vi "mainSynchro_PIV_LAT_translation.vi"() -> ()   [LabVIEW 2023]
uses:
  sousVis/configUtilisateur.ctl
  sousVis/customParam.ctl
  sousVis/configFPGA.ctl
  sousVis/defaultParam.ctl
  <vilib>/Instr/_visa.llb/VISA Configure Serial Port (Instr).vi
panel:
  in  "Home":bool
  in  "Tab Control":T1(tab)
  in  "TestComMoteur":bool
  in  "ComControler":refnum<visa-resource-name> caption="Port Com contrôleur"
  in  "ComMoteur":refnum<visa-resource-name> caption="Port Com moteur translation"
  in  "WriteConf":bool
  in  "readConf":bool
  in  "Configuration Moteurs":T2
  in  "Configuration contrôleur":T3={"Nombre de période"=0, "Fréquence "=10, "Nb pulse préchauffe laser"=0, "skip_frame_PIV"=0, "skip_frame_LAT"=0, "Time beetwen pulses (µs)"=10000, "Temps LAT (µs)"=20000, "Temps expo LAT (µs)"=10000, "action"=enum."PIV"}
  in  "customParam":T4={"CamDelayToOpen(µs)"=10, "FLWidth(µs)"=10, "QSWidth(µs)"=10, "DelayFL_QS (µs)"=180, "CamDelayToClose(µs)"=100, "CamPivExposure(µs)"=100}
  in  "StopPIV":bool
  in  "Play Button":bool
  out "XY Graph":cluster{cluster{"t_periode":i32, dbl}[]}[](graph)
  out "error out":errorcluster
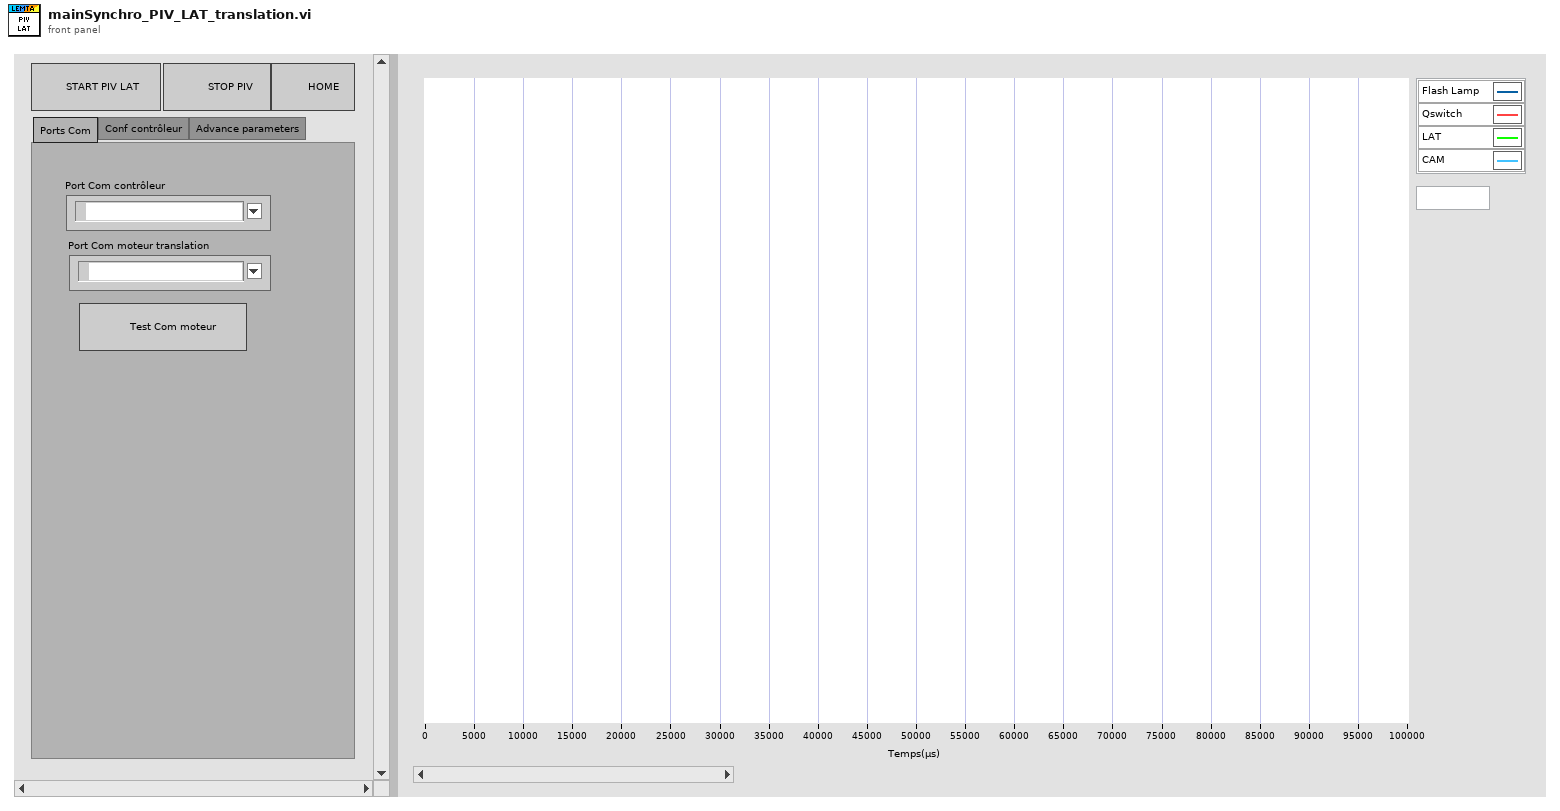
[diagram p1: front panel]
types:
  T1 = enum32{"Ports Com", "Conf contrôleur", "Advance parameters"}
  T2 = cluster{"Délais démarrage (ms)":dbl, "Vitesse (mm/s)":dbl, "Déplacement (mm)":dbl}
  T3 = typedef "configUtilisateur.ctl" = cluster{"Nombre de période":u16, "Fréquence ":u16, "Nb pulse préchauffe laser":u16, "skip_frame_PIV":u8, "skip_frame_LAT":u8, "Time beetwen pulses (µs)":u32, "Temps LAT (µs)":u32, "Temps expo LAT (µs)":u32, "action":enum8{"PIV", "PIV + LAT", "LAT"}}
  T4 = typedef "customParam.ctl" = cluster{"CamDelayToOpen(µs)":u32, "FLWidth(µs)":u32, "QSWidth(µs)":u32, "DelayFL_QS (µs)":u32, "CamDelayToClose(µs)":u32, "CamPivExposure(µs)":u32}
  T5 = typedef "configFPGA.ctl" = cluster{"action":enum8{"PIV", "PIV + LAT", "LAT", "STOP"}, "nb_periodes":u16, "t_periode":u32, "nb_pulse_prechauffe":u8, "nb_skip_frame_PIV":u8, "nb_skip_frame_LAT":u8, "t_FL1_start":u32, "t_FL1_stop":u32, "t_QS1_start":u32, "t_QS1_stop":u32, "t_FL2_start":u32, "t_FL2_stop":u32, "t_QS2_start":u32, "t_QS2_stop":u32, "t_LAT_start":u32, "t_LAT_stop":u32, "t_FRAME1_start":u32, "t_FRAME1_stop":u32, "t_FRAME2_start":u32, "t_FRAME2_stop":u32}
  T6 = typedef "defaultParam.ctl" = cluster{"customParam":T4, "Configuration":T3}
  T7 = cluster{"temps attente (ms)":i32, "vitesse (mm/s)":dbl, "Distance (mm)":dbl}
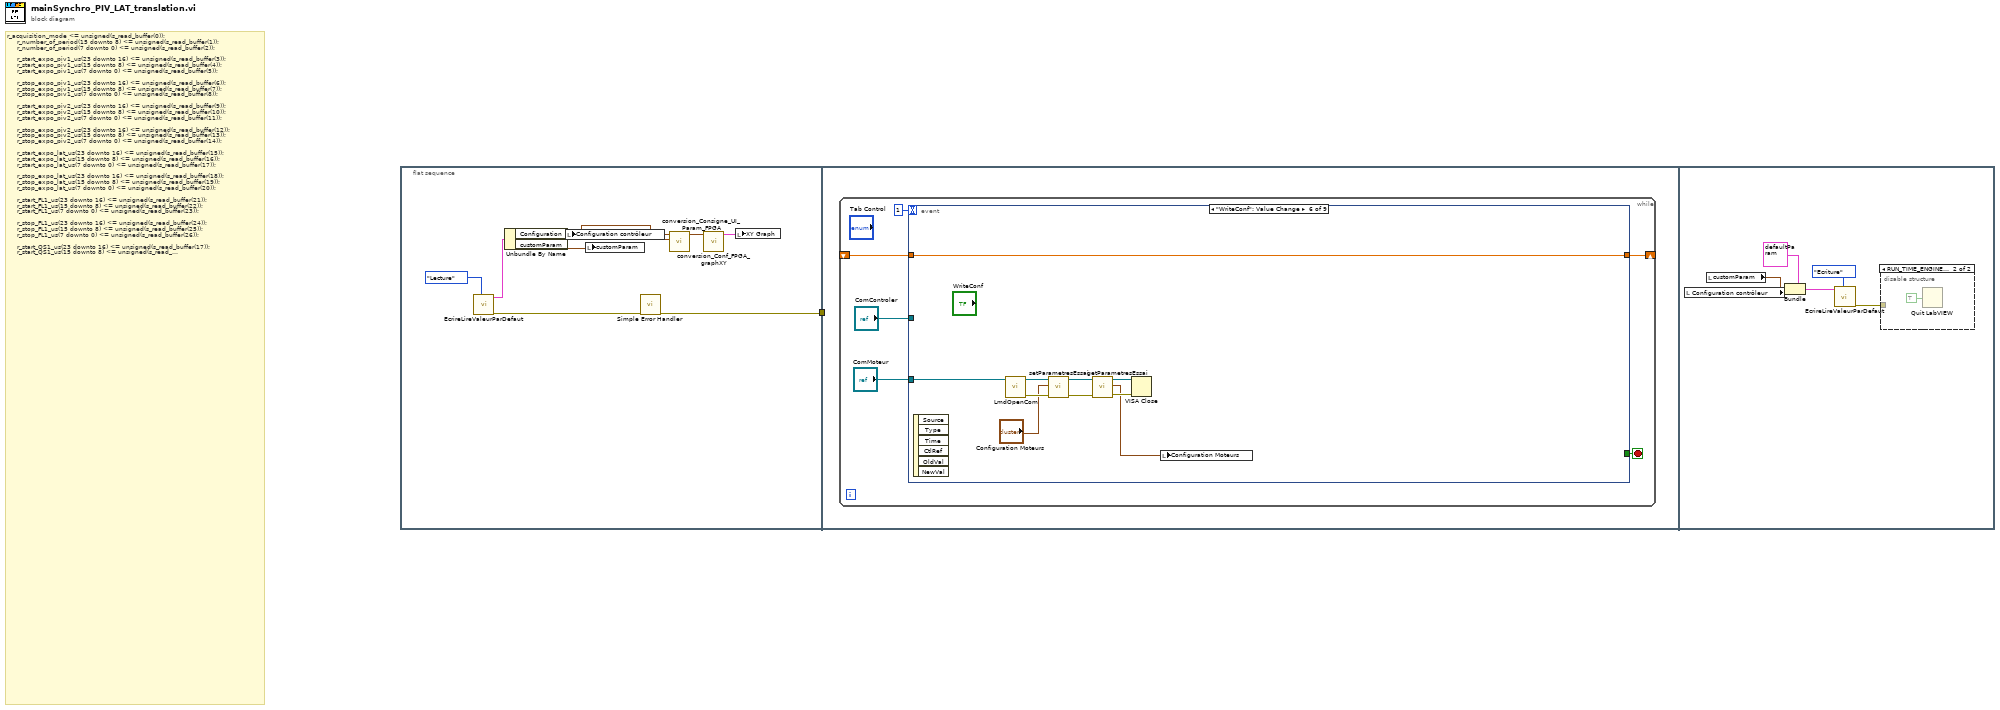
[diagram p0: block diagram]
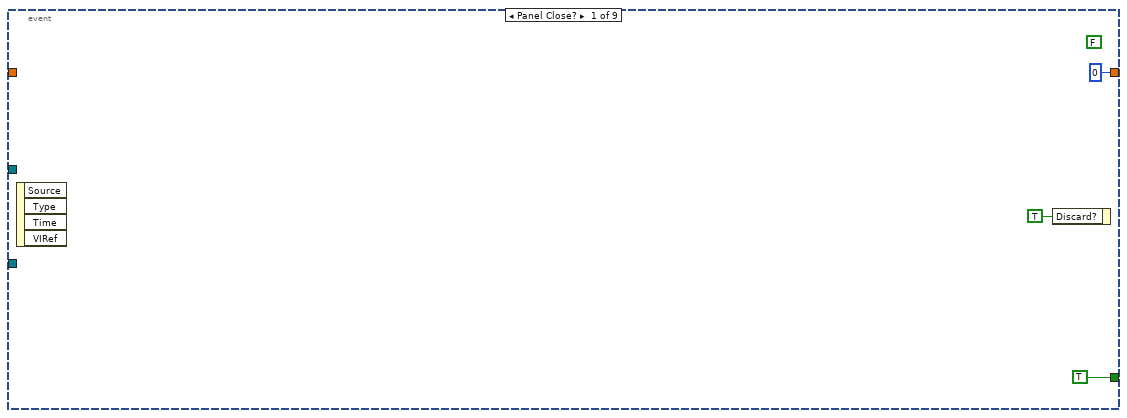
[diagram p2: hidden frame]
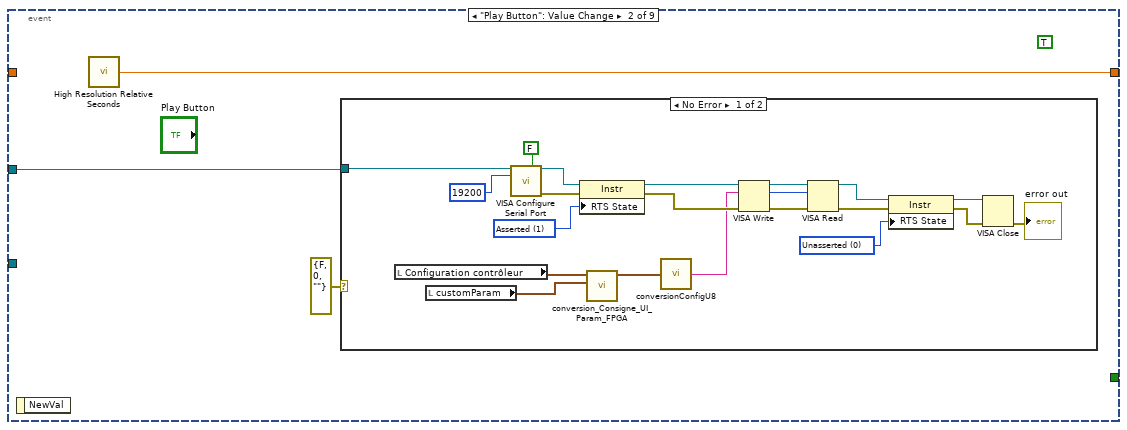
[diagram p3: hidden frame]
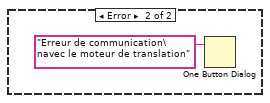
[diagram p4: hidden frame]
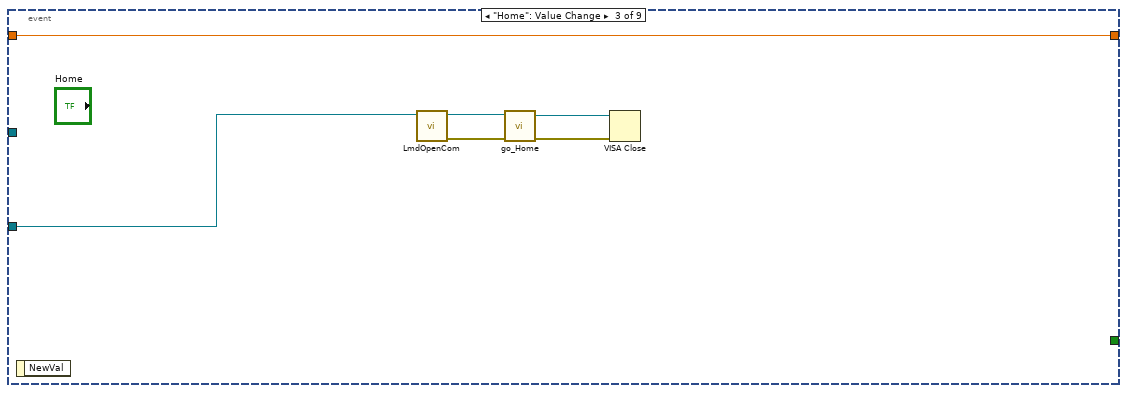
[diagram p5: hidden frame]
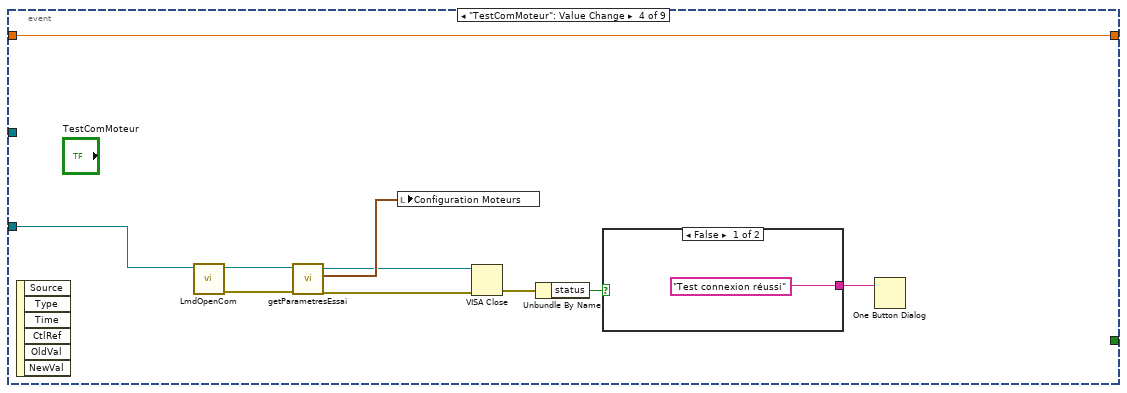
[diagram p6: hidden frame]
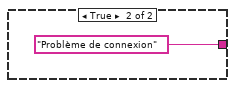
[diagram p7: hidden frame]
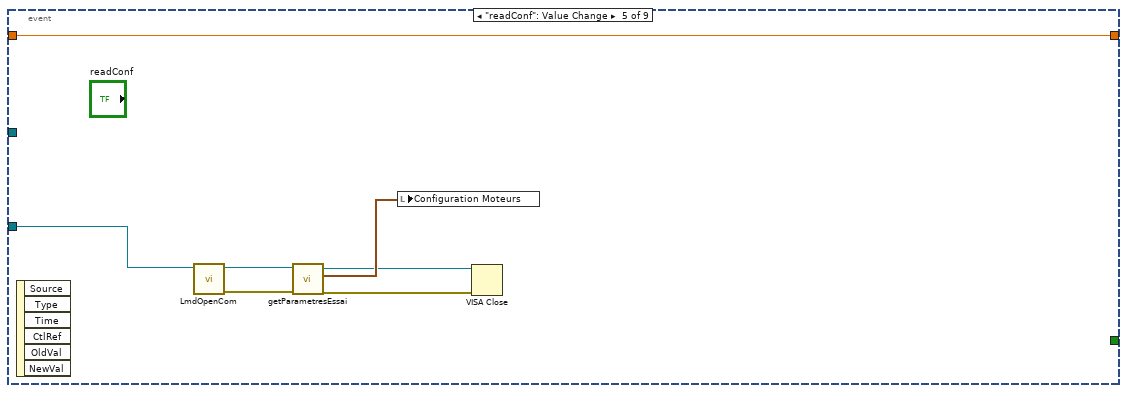
[diagram p8: hidden frame]
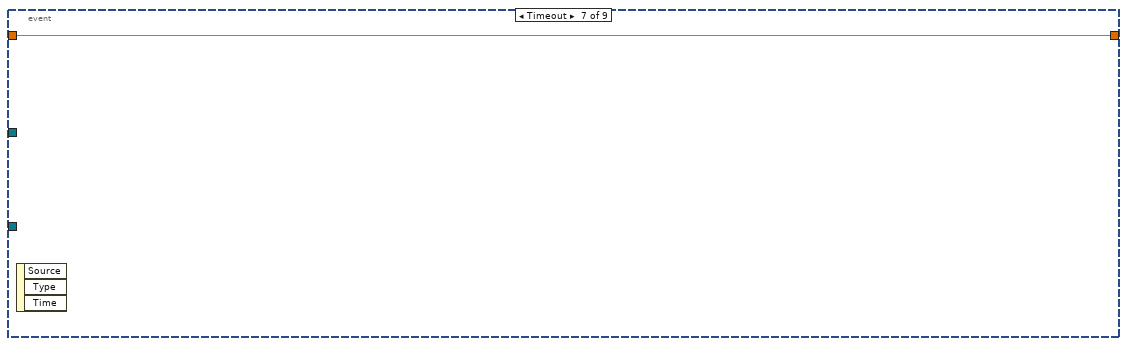
[diagram p9: hidden frame]
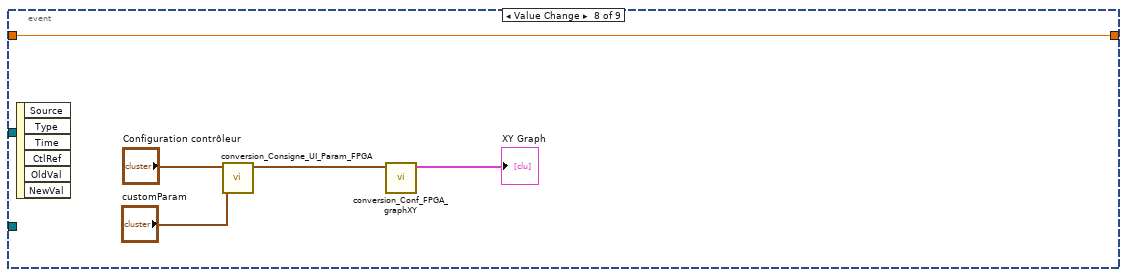
[diagram p10: hidden frame]
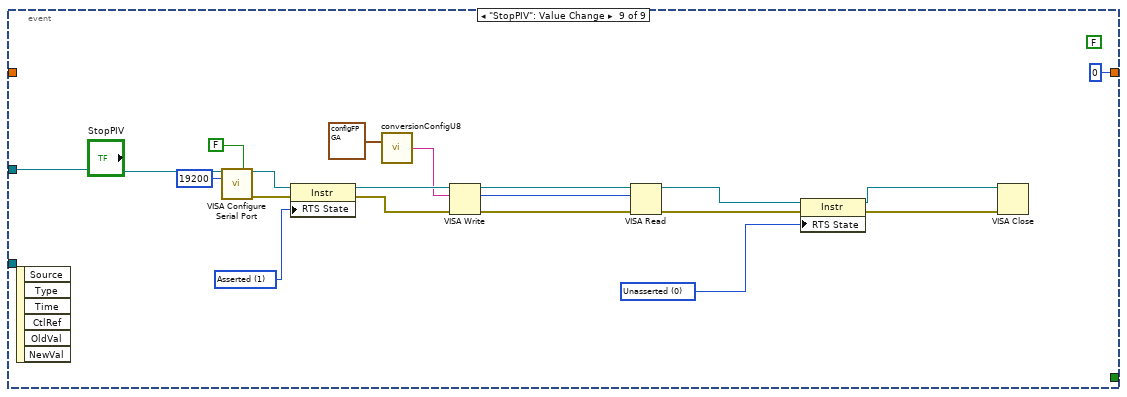
[diagram p11: hidden frame]
diagram:
  # "r_acquisition_mode <= unsigned(s_read_buffer(0));\n     r_number_of_period(15 downto 8) <= unsigned(s_read_buffer(1));\n\t\t\t\t\tr_number_of_period(7 downto 0) <= unsigned(s_read_buffer(2));\n\t\t\t\t\t\n\t\t\t\t\tr_start_expo_piv1_us(23 downto 16) <= unsigned(s_read_buffer(3));\n\t\t\t\t\tr_start_expo_piv1_us(15 downto 8) <= unsigned(s_read_buffer(4));\n\t\t\t\t\tr_start_expo_piv1_us(7 downto 0) <= unsigned(s_read_buffer(5));\n\t\t\t\t\t\n\t\t\t\t\tr_stop_expo_piv1_us(23 downto 16) <= unsigned(s_read_buffer(6));\n\t\t\t\t\tr_stop_expo_piv1_us(15 downto 8) <= unsigned(s_read_buffer(7));\n\t\t\t\t\tr_stop_expo_piv1_us(7 downto 0) <= unsigned(s_read_buffer(8));\n\t\t\t\t\t\n\t\t\t\t\tr_start_expo_piv2_us(23 downto 16) <= unsigned(s_read_buffer(9));\n\t\t\t\t\tr_start_expo_piv2_us(15 downto 8) <= unsigned(s_read_buffer(10));\n\t\t\t\t\tr_start_expo_piv2_us(7 downto 0) <= unsigned(s_read_buffer(11));\n\t\t\t\t\t\n\t\t\t\t\tr_stop_expo_piv2_us(23 downto 16) <= unsigned(s_read_buffer(12));\n\t\t\t\t\tr_stop_expo_piv2_us(15 downto 8) <= unsigned(s_read_buffer(13));\n\t\t\t\t\tr_stop_expo_piv2_us(7 downto 0) <= unsigned(s_read_buffer(14));\n\t\t\t\t\t\n\t\t\t\t\tr_start_expo_lat_us(23 downto 16) <= unsigned(s_read_buffer(15));\n\t\t\t\t\tr_start_expo_lat_us(15 downto 8) <= unsigned(s_read_buffer(16));\n\t\t\t\t\tr_start_expo_lat_us(7 downto 0) <= unsigned(s_read_buffer(17));\n\t\t\t\t\t\n\t\t\t\t\tr_stop_expo_lat_us(23 downto 16) <= unsigned(s_read_buffer(18));\n\t\t\t\t\tr_stop_expo_lat_us(15 downto 8) <= unsigned(s_read_buffer(19));\n\t\t\t\t\tr_stop_expo_lat_us(7 downto 0) <= unsigned(s_read_buffer(20));\n\t\t\t\t\t\n\t\t\t\t\tr_start_FL1_us(23 downto 16) <= unsigned(s_read_buffer(21));\n\t\t\t\t\tr_start_FL1_us(15 downto 8) <= unsigned(s_read_buffer(22));\n\t\t\t\t\tr_start_FL1_us(7 downto 0) <= unsigned(s_read_buffer(23));\n\t\t\t\t\t\n\t\t\t\t\tr_stop_FL1_us(23 downto 16) <= unsigned(s_read_buffer(24));\n\t\t\t\t\tr_stop_FL1_us(15 downto 8) <= unsigned(s_read_buffer(25));\n\t\t\t\t\tr_stop_FL1_us(7 downto 0) <= unsigned(s_read_buffer(26));\n\t\t\t\t\t\n\t\t\t\t\tr_start_QS1_us(23 downto 16) <= unsigned(s_read_buffer(17));\n\t\t\t\t\tr_start_QS1_us(15 downto 8) <= unsigned(s_read_buffer(28));\n\t\t\t\t\tr_start_QS1_us(7 downto 0) <= unsigned(s_read_buffer(29));\n\t\t\t\t\t\n\t\t\t\t\tr_stop_QS1_us(23 downto 16) <= unsigned(s_read_buffer(30));\n\t\t\t\t\tr_stop_QS1_us(15 downto 8) <= unsigned(s_read_buffer(31));\n\t\t\t\t\tr_stop_QS1_us(7 downto 0) <= unsigned(s_read_buffer(32));\n\t\t\t\t\t\n\t\t\t\t\tr_start_FL2_us(23 downto 16) <= unsigned(s_read_buffer(33));\n\t\t\t\t\tr_start_FL2_us(15 downto 8) <= unsigned(s_read_buffer(34));\n\t\t\t\t\tr_start_FL2_us(7 downto 0) <= unsigned(s_read_buffer(35));\n\t\t\t\t\t\n\t\t\t\t\tr_stop_FL2_us(23 downto 16) <= unsigned(s_read_buffer(36));\n\t\t\t\t\tr_stop_FL2_us(15 downto 8) <= unsigned(s_read_buffer(37));\n\t\t\t\t\tr_stop_FL2_us(7 downto 0) <= unsigned(s_read_buffer(38));\n\t\t\t\t\t\n\t\t\t\t\tr_start_QS2_us(23 downto 16) <= unsigned(s_read_buffer(39));\n\t\t\t\t\tr_start_QS2_us(15 downto 8) <= unsigned(s_read_buffer(40));\n\t\t\t\t\tr_start_QS2_us(7 downto 0) <= unsigned(s_read_buffer(41));\n\t\t\t\t\t\n\t\t\t\t\tr_stop_QS2_us(23 downto 16) <= unsigned(s_read_buffer(42));\n\t\t\t\t\tr_stop_QS2_us(15 downto 8) <= unsigned(s_read_buffer(43));\n\t\t\t\t\tr_stop_QS2_us(7 downto 0) <= unsigned(s_read_buffer(44));\n\t\t\t\t\t\n\t\t\t\t\tw_i_period_us(23 downto 16) <= unsigned(s_read_buffer(45));\n\t\t\t\t\tw_i_period_us(15 downto 8) <= unsigned(s_read_buffer(46));\n\t\t\t\t\tw_i_period_us(7 downto 0) <= unsigned(s_read_buffer(47));\n\t\t\t\t\t\n\t\t\t\t\tr_number_pulse_heat_laser(7 downto 0) <= unsigned(s_read_buffer(48));\n\t\t\t\t\t\n\t\t\t\t\tr_PIV_skip_frames(7 downto 0) <= unsigned(s_read_buffer(49));\n\t\t\t\t\t\n\t\t\t\t\tr_LAT_skip_frames(7 downto 0) <= unsigned(s_read_buffer(50));"
  n1 = flat-sequence {
    tunnel: [w2] -> w1
    tunnel: w1 -> [_]
    frame #0 {
      n2 = call "EcrireLireValeurParDefaut.vi"("Lecture/Ecriture"=enum32{"Lecture", "Ecriture"}."Lecture") -> ("error out"=w3:errorcluster, "defParametersOUT"=w8:T6)  [unwired: 8 in, 1 out]
      n3 = Unbundle By Name(w8) -> ("Configuration"=w7:T3, "customParam"=w6:T4)
      n4 = local write "Configuration contrôleur"(w7) -> ()
      n5 = local write "customParam"(w6) -> ()
      n6 = call <vilib>:"Simple Error Handler.vi"("error in (no error)"=w3) -> ("error out"=w2:errorcluster)  [unwired: 4 in, 4 out]
      n7 = call "conversion_Consigne_UI_Param_FPGA.vi"("customParam"=w6, "Config UI"=w7) -> ("Config FPGA"=w5:T5)  [unwired: 9 in]
      n8 = call "conversion_Conf_FPGA_graphXY.vi"("Config FPGA"=w5) -> ("appended array"=w4:cluster{cluster{"t_periode":i32, dbl}[]}[])  [unwired: 10 in]
      n9 = local write "XY Graph"(w4) -> ()
    }
    frame #1 {
      n10 = while {
        shift-right: [w12] -> _
        shift-left: _ -> [w11]
        stop <- w15 stop-if-true
        n11 = event shown="[5] \"WriteConf\": Value Change" {
          selector: _ -> [_ _ _ _ _ _ _ _ _]
          dyn-events: _ -> [_ _ _ _ _ _ _ _ _]
          timeout: 1 -> [_ _ _ _ _ _ _ _ _]
          tunnel: [TRUE _ _ _ _ _ _ _ _] -> w15
          tunnel: "ComControler" -> [_ w21 _ _ _ _ _ _ w89]
          tunnel: [u32 0 ("millisecond timer value") w20 w48 w50 w62 w78 w79 w80 u32 0 ("millisecond timer value")] -> w12
          tunnel: w11 -> [_ _ w48 w50 w62 w78 w79 w80 _]
          tunnel: "ComMoteur" -> [_ _ w49 w59 w68 w69 _ _ _]
          event Panel Close? {
            (unwired) FALSE
            n12 = event-data() -> ()  [unwired: 1 in, 4 out]
            n13 = event-data("Discard?"=TRUE) -> ()  [unwired: 1 in, 1 out]
          }
          event "Play Button": Value Change {
            (unwired) TRUE
            n14 = event-data() -> ()  [unwired: 1 in, 1 out]
            n15 = call <vilib>:"High Resolution Relative Seconds.vi"() -> ("relative seconds"=w20:dbl)
            n16 = case shown="No Error" errorcluster {"status"=FALSE, "code"=0, "source"=""} ("error IO") {
              tunnel: w21 -> [w27 _]
              frame No Error {
                w35 = i16 0 items=["Unknown"=-1, "Unasserted"=0, "Asserted"=1] ("Serial Settings:Modem Line Settings:Line RTS State")
                w41 = i16 1 items=["Unknown"=-1, "Unasserted"=0, "Asserted"=1] ("Serial Settings:Modem Line Settings:Line RTS State")
                n17 = local read "Configuration contrôleur"() -> (w24:T3)
                n18 = local read "customParam"() -> (w23:T4)
                n19 = call-poly "VISA Configure Serial Port"("VISA resource name"=w27, "Enable Termination\nChar (T)"=FALSE ("Enable Termination\nChar (T)"), "baud rate (9600)"=u32 19200) -> ("VISA resource name out"=w40:refnum<visa-resource-name>, "error out"=w39:errorcluster)  [unwired: 11 in]
                n20 = property class="Instr"(reference=w40, error in=w39, "RTS State"=w41) -> (reference out=w38:refnum<visa-resource-name>, error out=w37:errorcluster)
                n21 = call "conversion_Consigne_UI_Param_FPGA.vi"("customParam"=w23, "Config UI"=w24) -> ("Config FPGA"=w25:T5)  [unwired: 9 in]
                n22 = call "conversionConfigU8.vi"("Config"=w25) -> ("TrameConsigne"=w22:string)
                n23 = VISA Write(VISA resource name=w38, write buffer=w22, error in (no error)=w37) -> (VISA resource name out=w33:refnum<visa-resource-name>, return count=w34:u32, error out=w26:errorcluster)
                n24 = VISA Read(VISA resource name=w33, byte count=w34, error in (no error)=w26) -> (VISA resource name out=w31:refnum<visa-resource-name>, error out=w32:errorcluster)  [unwired: 2 out]
                n25 = property class="Instr"(reference=w31, error in=w32, "RTS State"=w35) -> (reference out=w30:refnum<visa-resource-name>, error out=w29:errorcluster)
                n26 = VISA Close(VISA resource name=w30, error in (no error)=w29) -> (error out=→"error out":errorcluster)
              }
              frame Error {
                n27 = One Button Dialog(message="Erreur de communication\navec le moteur de translation") -> ()  [unwired: 1 in, 1 out]
              }
            }
          }
          event "Home": Value Change {
            n28 = event-data() -> ()  [unwired: 1 in, 1 out]
            n29 = call "LmdOpenCom.vi"("VISA Refnum in"=w49) -> ("error out"=w46:errorcluster, "VISA Refnum out"=w47:refnum<visa-resource-name>)  [unwired: 9 in]
            n30 = call "go_Home.vi"("error in (no error)"=w46, "VISA resource name"=w47) -> ("error out"=w45:errorcluster, "VISA resource name out"=w44:refnum<visa-resource-name>)  [unwired: 8 in]
            n31 = VISA Close(VISA resource name=w44, error in (no error)=w45) -> ()  [unwired: 1 out]
          }
          event "TestComMoteur": Value Change {
            n32 = event-data() -> ()  [unwired: 1 in, 6 out]
            n33 = call "LmdOpenCom.vi"("VISA Refnum in"=w59) -> ("error out"=w54:errorcluster, "VISA Refnum out"=w58:refnum<visa-resource-name>)  [unwired: 9 in]
            n34 = call "getParametresEssai.vi"("error in (no error)"=w54, "VISA resource name"=w58) -> ("error out"=w55:errorcluster, "param out"=w57:T7, "VISA resource name out"=w56:refnum<visa-resource-name>)  [unwired: 7 in]
            n35 = local write "Configuration Moteurs"(w57) -> ()
            n36 = VISA Close(VISA resource name=w56, error in (no error)=w55) -> (error out=w53:errorcluster)
            n37 = Unbundle By Name(w53) -> ("status"=w52:bool)
            n38 = case shown="False" w52 {
              tunnel: ["Test connexion réussi" ("message") "Problème de connexion" ("message")] -> w51
              frame False {
              }
              frame True {
              }
            }
            n39 = One Button Dialog(message=w51) -> ()  [unwired: 1 in, 1 out]
          }
          event "readConf": Value Change {
            n40 = event-data() -> ()  [unwired: 1 in, 6 out]
            n41 = call "LmdOpenCom.vi"("VISA Refnum in"=w68) -> ("error out"=w63:errorcluster, "VISA Refnum out"=w67:refnum<visa-resource-name>)  [unwired: 9 in]
            n42 = call "getParametresEssai.vi"("error in (no error)"=w63, "VISA resource name"=w67) -> ("error out"=w64:errorcluster, "param out"=w66:T7, "VISA resource name out"=w65:refnum<visa-resource-name>)  [unwired: 7 in]
            n43 = local write "Configuration Moteurs"(w66) -> ()
            n44 = VISA Close(VISA resource name=w65, error in (no error)=w64) -> ()  [unwired: 1 out]
          }
          event "WriteConf": Value Change {
            n45 = event-data() -> ()  [unwired: 1 in, 6 out]
            n46 = call "LmdOpenCom.vi"("VISA Refnum in"=w69) -> ("error out"=w76:errorcluster, "VISA Refnum out"=w77:refnum<visa-resource-name>)  [unwired: 9 in]
            n47 = call "setParametresEssai.vi"("error in (no error)"=w76, "param"="Configuration Moteurs", "VISA resource name"=w77) -> ("error out"=w74:errorcluster, "VISA resource name out"=w75:refnum<visa-resource-name>)  [unwired: 7 in]
            n48 = call "getParametresEssai.vi"("error in (no error)"=w74, "VISA resource name"=w75) -> ("error out"=w72:errorcluster, "param out"=w70:T7, "VISA resource name out"=w71:refnum<visa-resource-name>)  [unwired: 7 in]
            n49 = VISA Close(VISA resource name=w71, error in (no error)=w72) -> ()  [unwired: 1 out]
            n50 = local write "Configuration Moteurs"(w70) -> ()
          }
          event Timeout {
            n51 = event-data() -> ()  [unwired: 1 in, 3 out]
          }
          event Value Change {
            n52 = event-data() -> ()  [unwired: 1 in, 6 out]
            n53 = call "conversion_Consigne_UI_Param_FPGA.vi"("customParam"="customParam", "Config UI"="Configuration contrôleur") -> ("Config FPGA"=w83:T5)  [unwired: 9 in]
            n54 = call "conversion_Conf_FPGA_graphXY.vi"("Config FPGA"=w83) -> ("appended array"=→"XY Graph":cluster{cluster{"t_periode":i32, dbl}[]}[])  [unwired: 10 in]
          }
          event "StopPIV": Value Change {
            (unwired) FALSE
            w97 = i16 0 items=["Unknown"=-1, "Unasserted"=0, "Asserted"=1] ("Serial Settings:Modem Line Settings:Line RTS State")
            w102 = i16 1 items=["Unknown"=-1, "Unasserted"=0, "Asserted"=1] ("Serial Settings:Modem Line Settings:Line RTS State")
            n55 = event-data() -> ()  [unwired: 1 in, 6 out]
            n56 = call-poly "VISA Configure Serial Port"("VISA resource name"=w89, "Enable Termination\nChar (T)"=FALSE ("Enable Termination\nChar (T)"), "baud rate (9600)"=u32 19200) -> ("VISA resource name out"=w101:refnum<visa-resource-name>, "error out"=w100:errorcluster)  [unwired: 11 in]
            n57 = property class="Instr"(reference=w101, error in=w100, "RTS State"=w102) -> (reference out=w99:refnum<visa-resource-name>, error out=w98:errorcluster)
            n58 = call "conversionConfigU8.vi"("Config"=T5 {"action"=enum."STOP", "nb_periodes"=0, "t_periode"=500000, "nb_pulse_prechauffe"=0, "nb_skip_frame_PIV"=0, "nb_skip_frame_LAT"=2, "t_FL1_start"=0, "t_FL1_stop"=100000, "t_QS1_start"=50000, "t_QS1_stop"=100000, "t_FL2_start"=100000, "t_FL2_stop"=200000, "t_QS2_start"=150000, "t_QS2_stop"=200000, "t_LAT_start"=300000, "t_LAT_stop"=400000, "t_FRAME1_start"=0, "t_FRAME1_stop"=100000, "t_FRAME2_start"=100000, "t_FRAME2_stop"=200000}) -> ("TrameConsigne"=w88:string)
            n59 = VISA Write(VISA resource name=w99, write buffer=w88, error in (no error)=w98) -> (VISA resource name out=w95:refnum<visa-resource-name>, return count=w96:u32, error out=w87:errorcluster)
            n60 = VISA Read(VISA resource name=w95, byte count=w96, error in (no error)=w87) -> (VISA resource name out=w93:refnum<visa-resource-name>, error out=w94:errorcluster)  [unwired: 2 out]
            n61 = property class="Instr"(reference=w93, error in=w94, "RTS State"=w97) -> (reference out=w92:refnum<visa-resource-name>, error out=w91:errorcluster)
            n62 = VISA Close(VISA resource name=w92, error in (no error)=w91) -> ()  [unwired: 1 out]
          }
        }
      }
    }
    frame #2 {
      n63 = local read "Configuration contrôleur"() -> (w106:T3)
      n64 = local read "customParam"() -> (w107:T4)
      n65 = Bundle(cluster=T6 {"customParam"={"CamDelayToOpen(µs)"=10, "FLWidth(µs)"=10, "QSWidth(µs)"=10, "DelayFL_QS (µs)"=180, "CamDelayToClose(µs)"=100, "CamPivExposure(µs)"=100}, "Configuration"={"Nombre de période"=2, "Fréquence "=0, "Nb pulse préchauffe laser"=41248, "skip_frame_PIV"=0, "skip_frame_LAT"=0, "Time beetwen pulses (µs)"=2, "Temps LAT (µs)"=0, "Temps expo LAT (µs)"=100000, "action"=enum."PIV + LAT"}} ("defParametersIN"), "customParam"=w107, "Configuration"=w106) -> (w105:T6)
      n66 = call "EcrireLireValeurParDefaut.vi"("Lecture/Ecriture"=enum32{"Lecture", "Ecriture"}."Ecriture", "defParametersIN"=w105) -> ("error out"=w104:errorcluster)  [unwired: 7 in, 2 out]
      n67 = disable-structure shown="RUN_TIME_ENGINE==True" {
        disable-tunnel: w104 -> [_ _]
        frame condition #0 (active) {
        }
        frame condition #1 {
          n68 = Quit LabVIEW(quit? (T)=TRUE) -> ()
        }
      }
    }
  }
